vi "Adjust to Deadzone.vi"(10 "Axis Value":dbl, 11 "Deadzone":dbl) -> (3 "Adjusted Axis Value":dbl)   [LabVIEW 2013]
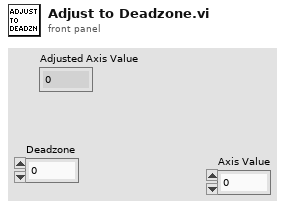
[diagram p1: front panel]
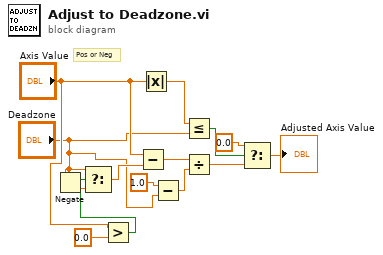
[diagram p0: block diagram]
diagram:
  # "Pos or Neg"
  n1 = Negate(x="Deadzone") -> (-x=w6:dbl)
  n2 = Greater?(x="Axis Value", y=0.0) -> (0:w3:bool)
  n3 = Select(t="Deadzone", s=w3, f=w6) -> (s? t:f=w2:dbl)
  n4 = Subtract(x="Axis Value", y=w2) -> (x-y=w9:dbl)
  n5 = Absolute Value(x="Axis Value") -> (abs(x)=w14:dbl)
  n6 = Subtract(x=1.0, y="Deadzone") -> (x-y=w10:dbl)
  n7 = Less Or Equal?(x=w14, y="Deadzone") -> (x <= y?=w13:bool)
  n8 = Divide(x=w9, y=w10) -> (x/y=w8:dbl)
  n9 = Select(t=0.0, s=w13, f=w8) -> (s? t:f=→"Adjusted Axis Value":dbl)
